vi "5.时间计数.vi"() -> ()   [LabVIEW 2019]
uses:
  <vilib>/rvi/Emulation/niFpgaGetClockAttributes.vi
  <vilib>/rvi/Emulation/niFpgaSctlEmulationGetInTimedLoop.vi
  <vilib>/rvi/Emulation/niFpgaEmulationReportErrorSimple.vi
  <vilib>/rvi/eio/common/nirviEmuTemplateMethod_errors.vi
  <vilib>/rvi/Emulation/niFpgaCriticalErrorInLSC.vi
  <vilib>/eio/EIONode/EIONode.xnode
panel:
  out "循环时间":u32
  out "Counters":u8
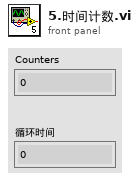
[diagram p1: front panel]
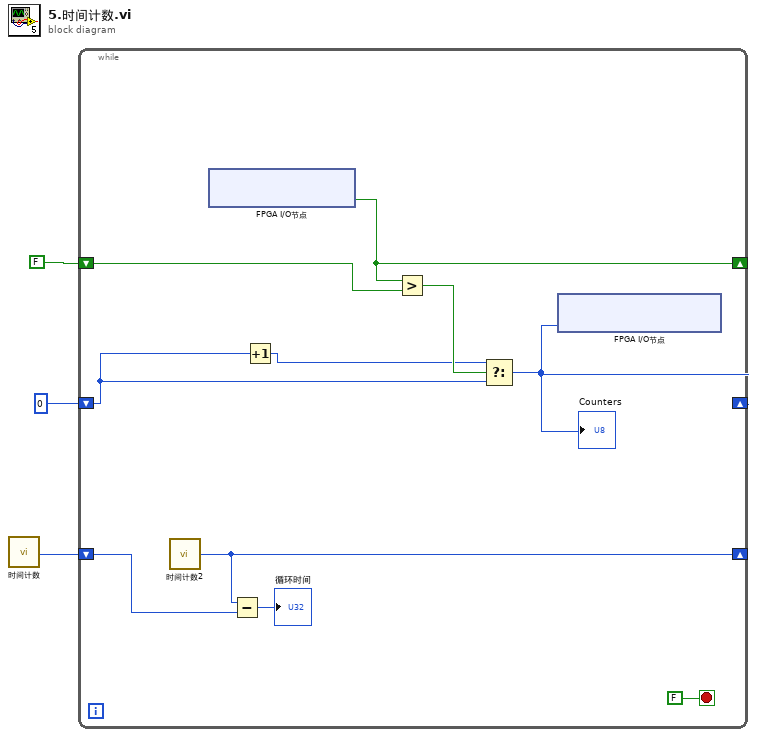
[diagram p0: block diagram]
diagram:
  n1 = call "时间计数"() -> ("Tick Count(Ticks)"=w1:u32)
  n2 = while {
    shift-right: [w11] -> _
    shift-left: FALSE -> [w12]
    shift-right: [w7] -> _
    shift-left: u8 0 -> [w8]
    shift-right: [w6] -> _
    shift-left: w1 -> [w5]
    stop <- FALSE stop-if-true
    n3 = call "时间计数2"() -> ("Tick Count(Ticks)"=w6:u32)
    n4 = xnode "FPGA I/O节点"() -> ("ConnectorA/DIO1"=w11:bool)  [unwired: 1 in, 1 out]
    n5 = Subtract(x=w6, y=w5) -> (x-y=→"循环时间":u32)
    n6 = Increment(x=w8) -> (x+1=w9:u8)
    n7 = Greater?(x=w11, y=w12) -> (0:w10:bool)
    n8 = Select(t=w9, s=w10, f=w8) -> (s? t:f=w7:u8)
    "Counters" <- w7
    n9 = xnode "FPGA I/O节点"("ConnectorA/DIO15:8"=w7) -> ()  [unwired: 1 in, 1 out]
  }
